vi "macro_NumCmd_Recv_Array.vi"() -> ()   [LabVIEW 2019, in "Trajectory_Library.lvlib"]
uses:
  VI/BoolCmd_Recv_Internal.vi
  VI/BoolCmd_ObtainQueue.vi
  Trajectory_Library.lvlib
panel:
  out "Values":dbl[](array[numeric])
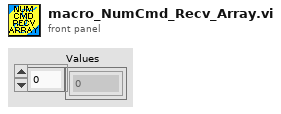
[diagram p1: front panel]
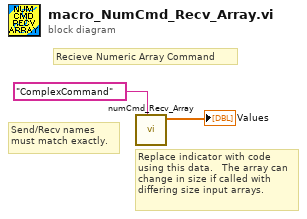
[diagram p0: block diagram]
diagram:
  # "Send/Recv names\nmust match exactly."
  # "Replace indicator with code\nusing this data.   The array can\nchange in size if called with \ndiffering size input arrays."
  # "Recieve Numeric Array Command"
  n1 = call "numCmd_Recv_Array.vi"("Command Name"="ComplexCommand") -> ("Values"=→"Values":dbl[])  [unwired: 8 in, 2 out]
